vi "Robot Global Data.vi"() -> ()   [LabVIEW 2018]
doc: "This global VI can contain as many global variables as you need. To create a global variable, place a control on the panel, give it a good name. To read or write to it from a VI, drag the icon to the diagram of that VI. You can also drag from the project. Click on the node to change which global you access. You shouldn't have multiple locations writing to a global or it will cause a race-condition."
uses:
  <vilib>/Rock Robotics/WPI/Camera/WPI_CameraImageSize.ctl
  <vilib>/Rock Robotics/WPI/DriverStation/WPI_DriverStationRobotMode2.ctl
  2018_Trobots_5013_Dashboard/Routines and Block Data.ctl
  2018_Trobots_5013_Robot/Support Code/Blocks.ctl
  <vilib>/Rock Robotics/WPI/MotorControl/WPI_MotorControlDeviceRef.ctl
  <vilib>/Rock Robotics/WPI/MotorControl/WPI_MotorControlType.ctl
  <vilib>/Rock Robotics/SystemInterfaces/DIO/FPGA_DIOPWMChannel.ctl
  <vilib>/Rock Robotics/WPI/PWM/WPI_PWMDeadband.ctl
  <vilib>/Rock Robotics/SystemInterfaces/DIO/FPGA_DIOChannel.ctl
panel:
  out "ms to process":u32
  out "Result":T1 {"Score" format="%#_3g"; "Pixels"."Rectangle"."Numeric 5" format="%#_3g"; "Pixels"."Rectangle"."Numeric 3" format="%#_3g"; "Pixels"."Rectangle"."Numeric 2" format="%#_3g"; "Pixels"."Rectangle"."Numeric" format="%#_3g"; "Normalized"."Rectangle"."Numeric 5" format="%#_2g"; "Normalized"."Rectangle"."Numeric 3" format="%#_2g"; "Normalized"."Rectangle"."Numeric 2" format="%#_2g"; "Normalized"."Rectangle"."Numeric" format="%#_2g"; "Normalized"."Center"."?" format="%#_3g"; "Normalized"."Center"."?" format="%#_3g"; "Distance (ft)" format="%#_3g"}
  in  "Pincher Enabled?":bool=TRUE
  in  "Elevator Enabled?":bool=TRUE
  in  "Intake Enabled?":bool=TRUE
  in  "Stop Motors":bool=TRUE
  in  "PhoenixMotorControlDevRef":T2={"DeviceStatus"={"status"=FALSE, "code"=0, "source"=""}, "Type"=enum."PWM", "PWM"={"PWM Channel"=enum."Invalid", "DeadBand"={"Name"="", "maxPositivePwm"=0, "minPositivePwm"=0, "centerPwm"=0, "maxNegativePwm"=0, "minNegativePwm"=0, "angularRange"=0}}, "CAN"={"Device Number"=0, "SetOutput VI Ref"=variant(refnum<vi> refnum), "GetOutput VI Ref"=variant(refnum<vi> refnum), "Enable VI Ref"=variant(refnum<vi> refnum), "Disable VI Ref"=variant(refnum<vi> refnum), "Data"=variant}, "Invert"=FALSE, "DIO PWM"={"PWM \"Enable\" Channel"=enum."Invalid", "DIOChannel"=enum."Invalid", "PWM Rate"=0.0}}
  in  "Routines and Block Data":T7
  in  "Gyro Refnum Ready":bool
  in  "Robot Mode":T9
  in  "image size":T10=enum."320x240"
  in  "Enable Vision":bool
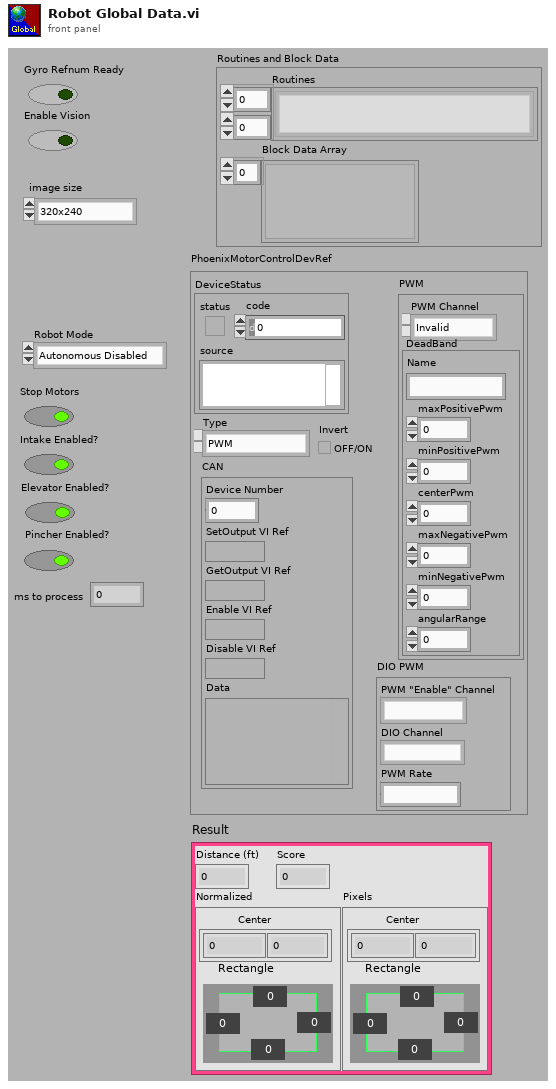
[diagram p1: front panel]
types:
  T1 = cluster{"Distance (ft)":dbl, "Score":dbl, "Normalized":cluster{"Center":cluster{dbl, dbl}, "Rectangle":cluster{"Numeric":dbl, "Numeric 2":dbl, "Numeric 3":dbl, "Numeric 5":dbl}}, "Pixels":cluster{"Center":cluster{dbl, dbl}, "Rectangle":cluster{"Numeric":dbl, "Numeric 2":dbl, "Numeric 3":dbl, "Numeric 5":dbl}}}
  T2 = typedef "WPI_MotorControlDeviceRef.ctl" = cluster{"DeviceStatus":errorcluster, "Type":T3, "PWM":cluster{"PWM Channel":T4, "DeadBand":T5}, "CAN":cluster{"Device Number":u8, "SetOutput VI Ref":variant, "GetOutput VI Ref":variant, "Enable VI Ref":variant, "Disable VI Ref":variant, "Data":variant}, "Invert":bool, "DIO PWM":cluster{"PWM \"Enable\" Channel":T4, "DIOChannel":T6, "PWM Rate":dbl}}
  T3 = typedef "WPI_MotorControlType.ctl" = enum16{"PWM", "CAN", "DIO PWM"}
  T4 = typedef "FPGA_DIOPWMChannel.ctl" = enum8{"PWM 0", "PWM 1", "PWM 2", "PWM 3", "PWM 4", "PWM 5", "PWM 6", "PWM 7", "PWM 8", "PWM 9", "PWM MXP 0", "PWM MXP 1", "PWM MXP 2", "PWM MXP 3", "PWM MXP 4", "PWM MXP 5", "PWM MXP 6", "PWM MXP 7", "PWM MXP 8", "PWM MXP 9", "Invalid"}
  T5 = typedef "WPI_PWMDeadband.ctl" = cluster{"Name":string, "maxPositivePwm":i32, "minPositivePwm":i32, "centerPwm":i32, "maxNegativePwm":i32, "minNegativePwm":i32, "angularRange":u16}
  T6 = typedef "FPGA_DIOChannel.ctl" = enum8{"DIO 0", "DIO 1", "DIO 2", "DIO 3", "DIO 4", "DIO 5", "DIO 6", "DIO 7", "DIO 8", "DIO 9", "DIO MXP 0", "DIO MXP 1", "DIO MXP 2", "DIO MXP 3", "DIO MXP 4", "DIO MXP 5", "DIO MXP 6", "DIO MXP 7", "DIO MXP 8", "DIO MXP 9", "DIO MXP 10", "DIO MXP 11", "DIO MXP 12", "DIO MXP 13", "DIO MXP 14", "DIO MXP 15", "SPI Port CS1", "SPI Port CS2", "SPI Port CS3", "SPI Port MISO", "SPI Port MOSI", "Invalid"}
  T7 = typedef "Routines and Block Data.ctl" = cluster{"Routines":T8[][], "Block Data Array":variant[]}
  T8 = typedef "Blocks.ctl" = enum16{"", "Wait 1s", "Far--L", "L--end Sw", "end Sw--sq C1", "end cube--C1", "C1--d Hi", "C1--C3", "C3--C4", "d Hi--C1", "C3--end Sw", "C3--cube Sw", "M--front LSw", "M--front RSw", "front Sw--L", "L--C1", "C1--end cube", "sq Hi--C1", "C1--sq Hi", "front Sw--P cube1", "P cube1--front Sw"}
  T9 = typedef "WPI_DriverStationRobotMode2.ctl" = enum16{"Autonomous Disabled", "Autonomous Enabled", "Teleop Disabled", "Teleop Enabled", "Disconnected", "Finish", "Test Disabled", "Test Enabled", "Emergency Stopped"}
  T10 = typedef "WPI_CameraImageSize.ctl" = enum16{"640x480", "320x240", "160x120", "Custom"}
diagram:
